vi "Write Resynchronize Microgrid Msg.vi"(10 "Resynchronize Microgrid Msg":refnum<class "Resynchronize Microgrid Msg.lvclass">, 11 "Remote Operation Abstract in":refnum<class "Remote Operation Abstract.lvclass">) -> (3 "Remote Operation Abstract out":refnum<class "Remote Operation Abstract.lvclass">)   [LabVIEW 2018, in "Remote Operation Abstract.lvlib" / "Remote Operation Abstract.lvclass"]
uses:
  Remote Operation Abstract.lvclass
  Remote Operation Abstract Messages/Resynchronize Microgrid Msg/Resynchronize Microgrid Msg.lvclass
  Remote Operation Abstract.lvclass/Remote Operation Abstract.ctl
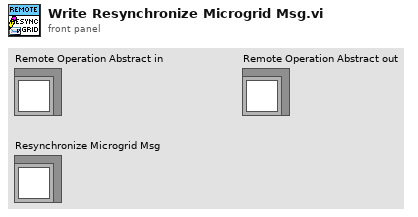
[diagram p1: front panel]
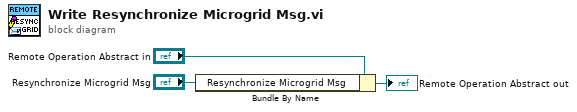
[diagram p0: block diagram]
diagram:
  n1 = Bundle By Name(cluster="Remote Operation Abstract in", "Resynchronize Microgrid Msg"="Resynchronize Microgrid Msg") -> (→"Remote Operation Abstract out":refnum<class "Remote Operation Abstract.lvclass">)
